vi "ЛР2 - 1 варик.vi"() -> ()   [LabVIEW 2012]
panel:
  in  "Slide 3":dbl(slide) scale=0.0..250.0
  in  "Slide 2":dbl(slide) scale=0.0..10.0
  out "Boolean 3":bool
  out "Waveform Chart 2":dbl(graph)
  in  "Dial 2":dbl(knob) scale=-10.0..10.0
  out "Boolean 4":bool
  out "Boolean 2":bool
  in  "Numeric 2":dbl
  in  "Numeric":dbl
  out "Meter":dbl(knob) scale=0.0..10.0
  out "Waveform Chart":dbl[](graph)
  in  "stop":bool
  in  "1":bool
  in  "Dial":dbl(knob) scale=-10.0..10.0
  in  "Slide":dbl(slide) scale=0.0..10.0
  # "2"
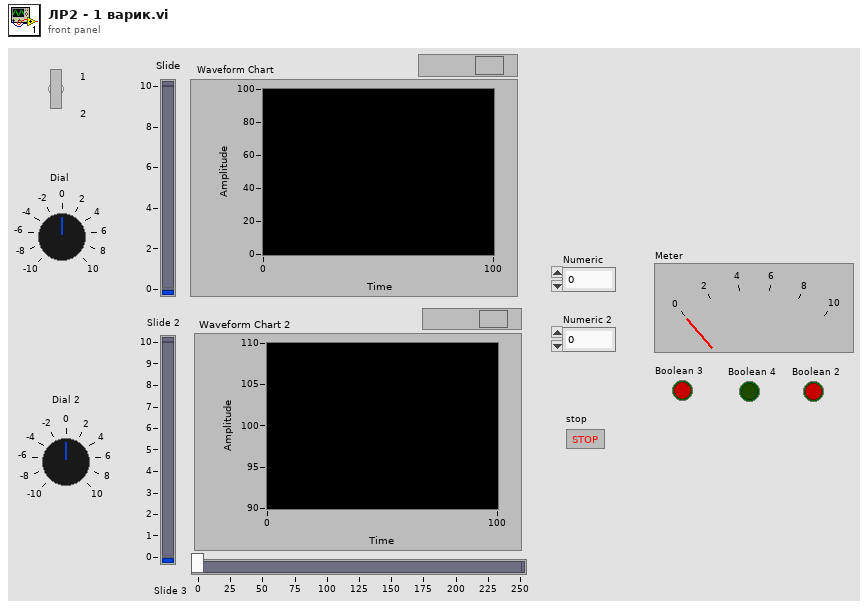
[diagram p1: front panel]
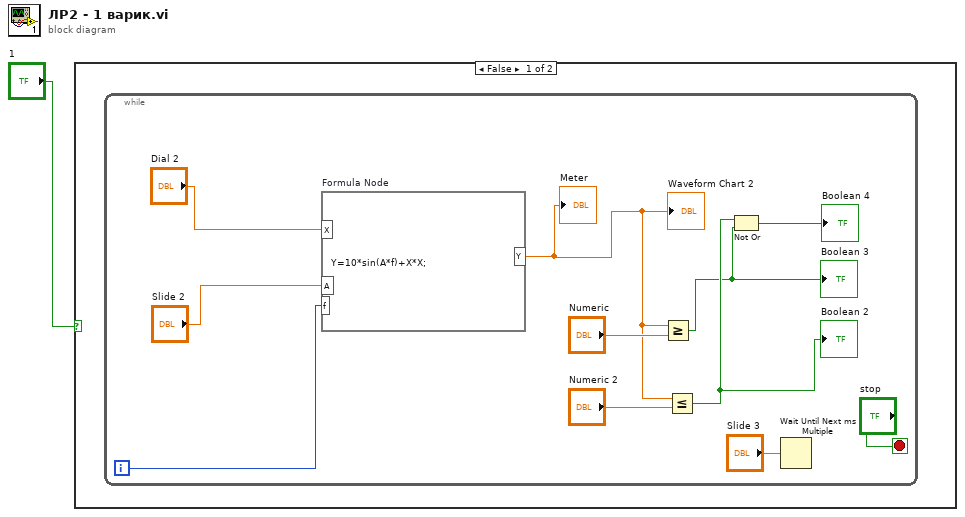
[diagram p0: block diagram]
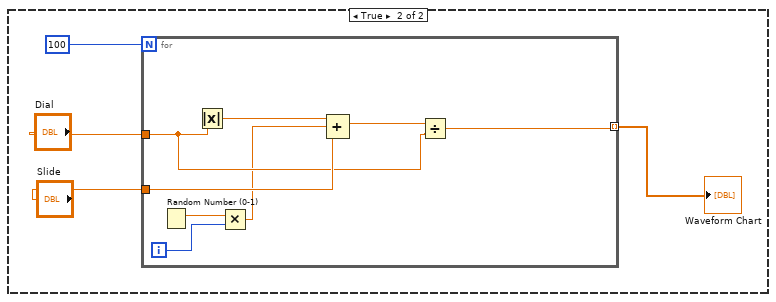
[diagram p2: hidden frame]
diagram:
  n1 = case shown="False" "1" {
    frame False {
      n2 = while {
        i -> [w6]
        stop <- "stop" stop-if-true
        n3 = formula code="Y=10*sin(A*f)+X*X;"("X"="Dial 2", "A"="Slide 2", "f"=w6) -> ("Y"=w3:dbl)
        "Meter" <- w3
        "Waveform Chart 2" <- w3
        n4 = Greater Or Equal?(x=w3, y="Numeric") -> (x >= y?=w2:bool)
        "Boolean 3" <- w2
        n5 = Less Or Equal?(x=w3, y="Numeric 2") -> (x <= y?=w4:bool)
        "Boolean 2" <- w4
        n6 = Not Or(1:w2, 2:w4) -> (0:→"Boolean 4":bool)
        n7 = Wait Until Next ms Multiple(millisecond multiple="Slide 3") -> ()  [unwired: 1 out]
      }
    }
    frame True {
      n8 = for {
        N: 100 -> [_]
        tunnel: "Slide" -> [w23]
        tunnel: "Dial" -> [w21]
        tunnel: [w20] -> w15 mode=indexing
        i -> [w18]
        n9 = Random Number (0-1)() -> (number: 0 to 1=w19:dbl)
        n10 = Absolute Value(x=w21) -> (abs(x)=w24:dbl)
        n11 = Multiply(x=w19, y=w18) -> (x*y=w17:dbl)
        n12 = Compound Arithmetic op=ADD(w24, w17, w23) -> (w22:dbl)
        n13 = Divide(x=w22, y=w21) -> (x/y=w20:dbl)
      }
      "Waveform Chart" <- w15
    }
  }
